vi "Write SelectedAxis.vi"(8 "error in (no error)":errorcluster, 10 "SelectedAxis":u32, 11 "Picomoto8742ControllerClass in":refnum<class "Picomoto8742ControllerClass.lvclass">) -> (0 "error out":errorcluster, 3 "Picomoto8742ControllerClass out":refnum<class "Picomoto8742ControllerClass.lvclass">)   [LabVIEW 2013, in "Picomoto8742ControllerClass.lvclass"]
uses:
  Picomoto8742ControllerClass.lvclass
  Picomoto8742ControllerClass.lvclass/Picomoto8742ControllerClass.ctl
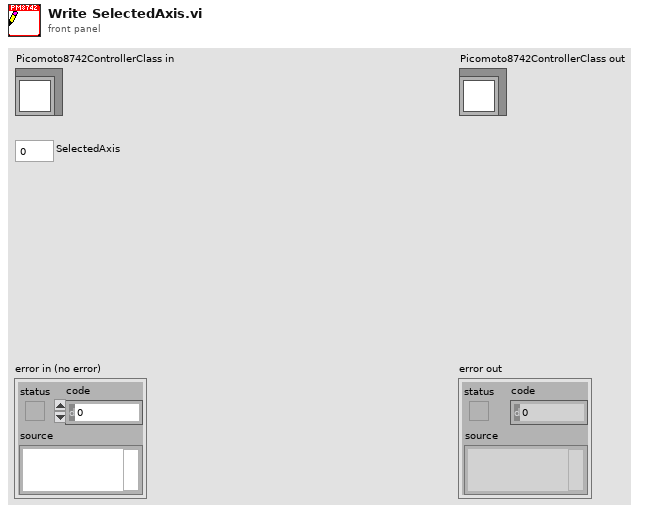
[diagram p1: front panel]
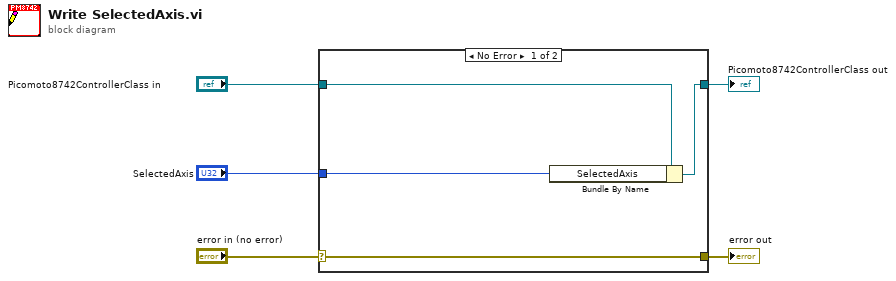
[diagram p0: block diagram]
diagram:
  n1 = case shown="No Error" "error in (no error)" {
    selector: "error in (no error)" -> [w9 w10]
    tunnel: [w9 w10] -> w4
    tunnel: [w7 w11] -> w2
    tunnel: "Picomoto8742ControllerClass in" -> [w8 w11]
    tunnel: "SelectedAxis" -> [w6 _]
    frame No Error {
      n2 = Bundle By Name(cluster=w8, "SelectedAxis"=w6) -> (w7:refnum<class "Picomoto8742ControllerClass.lvclass">)
    }
    frame Error {
    }
  }
  "error out" <- w4
  "Picomoto8742ControllerClass out" <- w2
